vi "Get Diagnostics.vi"(8 "error in (no error)":errorcluster, 11 "Temperature Controller in":refnum<class "Temperature Controller.lvclass">) -> (0 "error out":errorcluster, 2 "Diagnostics":string, 3 "Temperature Controller out":refnum<class "Temperature Controller.lvclass">)   [LabVIEW 2024, in "Temperature Controller.lvclass"]
uses:
  Temperature Controller.lvclass
  C:/Git/LabActor/Template Module/Template Module.lvclass
  C:/Program Files/National Instruments/LabVIEW 2024/vi.lib/ActorFramework/Actor/Actor.lvclass
  NHMFL_Core/Libraries/Instruments/Results/String Result/String Result.lvclass
  C:/Git/LabActor/Publish-Subscribe/Interfaces/Information/Information.lvclass
  Template Module/Template Module.lvclass/Template Module.ctl
  <vilib>/ActorFramework/Actor/Actor.lvclass/Actor.ctl
  Publish-Subscribe/Interfaces/Subscriber Messages/Information Msg/Information Msg.lvclass/Information Msg.ctl
  <vilib>/ActorFramework/Message Enqueuer/Message Enqueuer.lvclass/Message Enqueuer.ctl
  Template Module/Read Name.vi
  <vilib>/ActorFramework/Message Enqueuer/Enqueue.vi
  Publish-Subscribe/Interfaces/Subscriber Messages/Information Msg/Information Msg.lvclass
  C:/Program Files/National Instruments/LabVIEW 2024/vi.lib/ActorFramework/Message/Message.lvclass
  <vilib>/ActorFramework/Message Priority Queue/Priority Enqueue.vi
  Continuous Recorder Actor/Continuous Recorder Actor.lvclass
  Temperature Controller.lvclass/Temperature Controller.ctl
  <vilib>/ActorFramework/Actor/Actor.lvclass
  C:/Git/LabActor/Recorders/Continuous Recorder Actor/Continuous Recorder Actor.lvclass
  C:/Git/LabActor/Instrument Actor/Instrument Actor.lvclass
  C:/Git/LabActor/Worker/Worker Actor/Worker Actor.lvclass
  C:/Git/LabActor/Worker/Woker Interface/Worker.lvclass
  C:/Git/LabActor/Recorders/Interfaces/Continuous Recorder/Continuous Recorder.lvclass
  C:/Git/LabActor/Recorders/Temperature Controller/Temperature Controller.lvclass
  C:/Git/NHMFL_Core/Libraries/Instruments/Results/Acquired Result/Acquired Result.lvclass
  C:/Git/NHMFL_Core/Libraries/Instruments/Results/String Result/String Result.lvclass
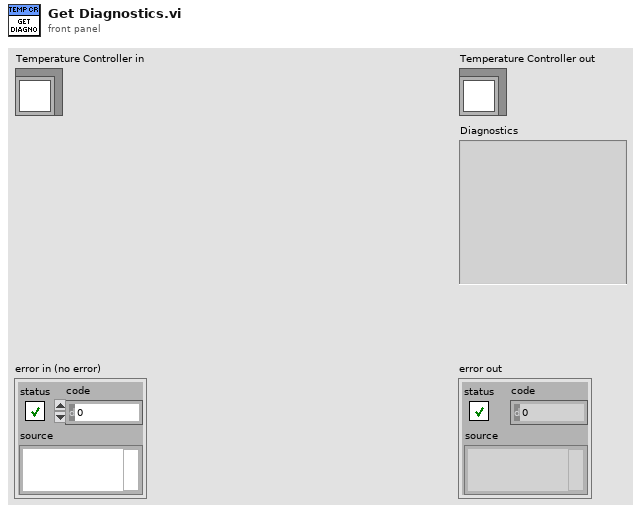
[diagram p1: front panel]
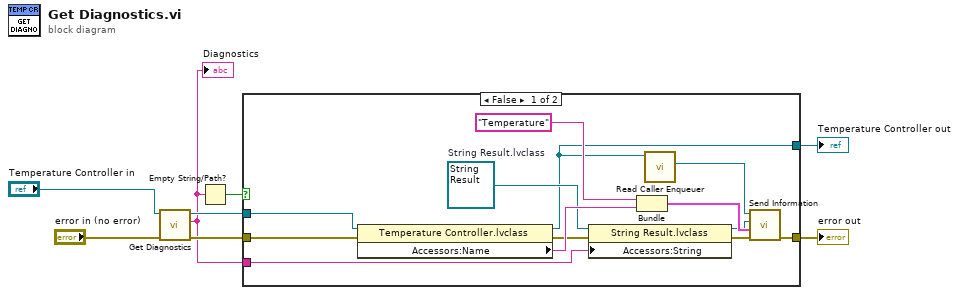
[diagram p0: block diagram]
diagram:
  n1 = call-parent "Get Diagnostics.vi"("error in (no error)"="error in (no error)", "Instrument Actor in"="Temperature Controller in") -> ("error out"=w5:errorcluster, "Diagnostics"=w4:string, "Instrument Actor out"=w6:refnum<class "Temperature Controller.lvclass">)  [unwired: 7 in]
  "Diagnostics" <- w4
  n2 = Empty String/Path?(string/path=w4) -> (empty?=w3:bool)
  n3 = case shown="False" w3 {
    tunnel: w6 -> [w21 w22]
    tunnel: w5 -> [w16 w23]
    tunnel: w4 -> [w14 _]
    tunnel: [w10 w23] -> w2
    tunnel: [w9 w22] -> w1
    frame False {
      w15 = refnum<class "String Result.lvclass"> refnum  # String Result.lvclass
      n4 = property class="Temperature Controller.lvclass"(reference=w21, error in=w16) -> (reference out=w9:refnum<class "Temperature Controller.lvclass">, error out=w12:errorcluster, "Accessors:Name"=w19:string)
      n5 = property class="String Result.lvclass"(reference=w15, error in=w12, "Accessors:String"=w14) -> (reference out=w13:refnum<class "String Result.lvclass">, error out=w11:errorcluster)
      n6 = Bundle("Temperature", "Accessors:Name"=w19) -> (w17:cluster{string, "Accessors:Name":string})  [unwired: 1 in]
      n7 = call <vilib>:"Read Caller Enqueuer.vi"("Actor"=w9) -> ("Caller Enqueuer"=w20:refnum<class "Message Enqueuer.lvclass">)  [unwired: 10 in]
      n8 = call "Send Information.vi"("error in (no error)"=w11, "Context"=w17, "Information"=w13, "Message Enqueuer"=w20) -> ("error out"=w10:errorcluster)  [unwired: 6 in, 1 out]
    }
    frame True {
    }
  }
  "error out" <- w2
  "Temperature Controller out" <- w1
